vi "ATF-Pump-DI_Read.vi"(8 "error in (no error)":errorcluster, 9 "number of samples per channel":i32, 10 "DI_Task":refnum<k21>, 11 "Data FIFO Ref":T1) -> (0 "error out":errorcluster, 2 "task out":refnum<k21>)   [LabVIEW 2022 SP3]
uses:
  RT Controls/ATF-Pump-Data FIFO.ctl
  <vilib>/Platform/TimedLoop/XDataNode/timing_clust.ctl
  <vilib>/Platform/TimedLoop/XDataNode/nitl_modes.ctl
  <vilib>/Platform/TimedLoop/XDataNode/wakeup.ctl
  <vilib>/DAQmx/read.llb/DAQmx Read (Digital 1D Wfm NChan NSamp).vi
  <vilib>/DAQmx/miscellaneous.llb/DAQmx Fill In Error Info.vi
  <vilib>/Waveform/DTblOps.llb/DTbl Digital to Boolean Array.vi
  <vilib>/platform/TimedLoop/XDataNode/XDataNode.xnode
  <vilib>/Platform/TimedLoop/XDataNode/XDNodeRunTimeDep.lvlib
panel:
  out "overflow?":bool
  out "x-y":u32
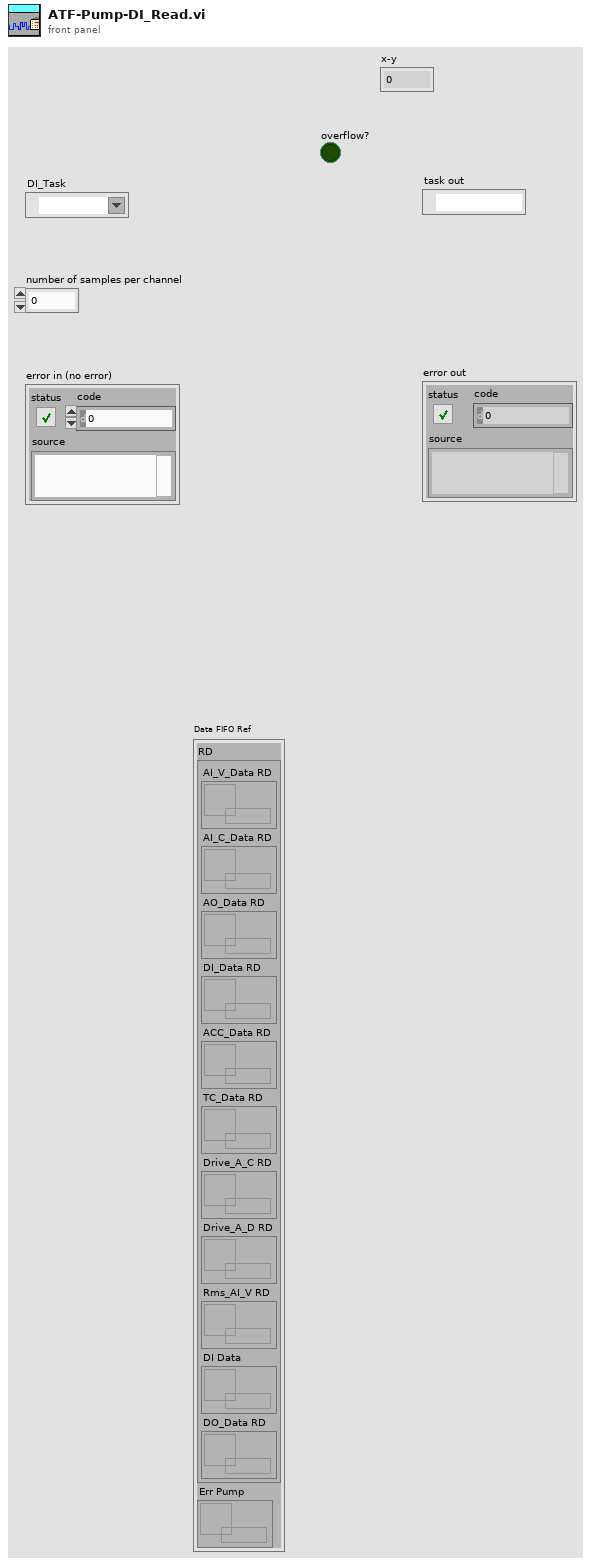
[diagram p1: front panel]
types:
  T1 = typedef "ATF-Pump-Data FIFO.ctl" = cluster{"RD":cluster{"AI_V_Data RD":refnum<queue>, "AI_C_Data RD":refnum<queue>, "AO_Data RD":refnum<queue>, "DI_Data RD":refnum<queue>, "ACC_Data RD":refnum<queue>, "TC_Data RD":refnum<queue>, "Drive_A_C RD":refnum<queue>, "Drive_A_D RD":refnum<queue>, "Rms_AI_V RD":refnum<queue>, "DI Data":refnum<queue>, "DO_Data RD":refnum<queue>}, "Err Pump":refnum<queue>}
  T2 = typedef "XDNodeRunTimeDep.lvlib/timing_clust.ctl" = cluster{"Expected End [f-1]":u64, "Actual End [f-1]":u64, "Finished Late? [f-1]":bool, "Expected End [i-1]":u64, "Actual End [i-1]":u64, "Finished Late? [i-1]":bool, "Expected Start [i]":u64, "Actual Start [i]":u64, "Expected Start [f]":u64, "Actual Start [f]":u64, "Source Name":string, "Structure Name":string, "Period":i64, "Deadline":i64, "Offset":i64, "Start":i64, "Priority":i32, "Timeout":i32, "Mode":T3, "Wakeup Reason":T4, "Error":errorcluster, "Source Type":string, "Secondary Source Type":string, "Global End Time":u64, "Global Start Time":u64, "Frame Duration":u64, "Iteration Duration":u64, "Assigned CPU":i32, "I/O Scan Engine Mode":u32}
  T3 = typedef "XDNodeRunTimeDep.lvlib/nitl_modes.ctl" = enum32{"No Change", "Process missed periods, maintain original phase", "Discard missed periods, maintain original phase", "Process missed periods, ignore original phase", "Discard missed periods, ignore original phase"}
  T4 = typedef "XDNodeRunTimeDep.lvlib/wakeup.ctl" = enum32{"Normal", "Aborted", "Asynchronous wakeup", "Timing source error", "Timed loop error", "Timeout"}
  T5 = enum16{"AI C", "AI V", "AO", "DI", "DO", "TC", "ACC", "RT PMP", "DR A"}
  T6 = enum16{"Init", "Read 'All'", "Read 'n'", "Read '1'", "Write '1'", "Write 'n'", "Write 'All'"}
  T7 = cluster{"Start DAQ":bool, "Stop DAQ":bool, "RT Stop":bool, "RT Exit":bool, "Start Seq":bool}
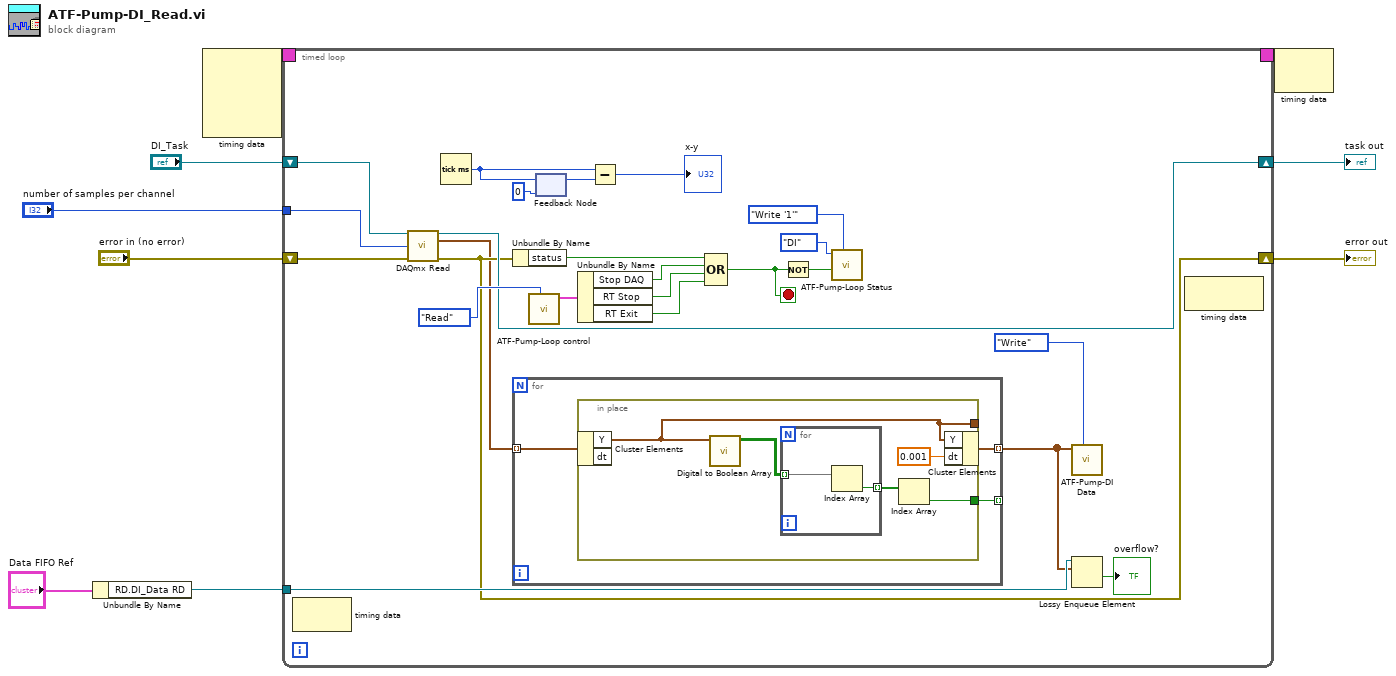
[diagram p0: block diagram]
diagram:
  n1 = Unbundle By Name("Data FIFO Ref") -> ("RD.DI_Data RD"=w3:refnum<queue>)
  n2 = node-c288() -> (w2:T2)  [unwired: 4 in]
  n3 = timed-loop {
    tunnel: "number of samples per channel" -> [w10]
    tunnel: w3 -> [w16]
    shift-right: [w18] -> w6
    shift-left: "DI_Task" -> [w32]
    shift-right: [w14] -> w5
    shift-left: "error in (no error)" -> [w31]
    timing: w2 -> [_]
    timing-out: [_] -> w1
    stop <- w33 stop-if-true
    n4 = node-c288() -> ()  [unwired: 1 in, 1 out]
    n5 = call-poly <vilib>:"DAQmx Read.vi"("task/channels in"=w32, "number of samples per channel"=w10, "error in"=w31) -> ("task out"=w18:refnum<k21>, "data"=w13:digitalwaveform[], "error out"=w14:errorcluster)  [unwired: 10 in]
    n6 = Tick Count (ms)() -> (millisecond timer value=w22:u32)
    n7 = Unbundle By Name(w14) -> ("status"=w30:bool)
    n8 = for {
      tunnel: w13 -> [w37] mode=indexing
      tunnel: [w38] -> _ mode=indexing
      tunnel: [w36] -> w12 mode=indexing
      n9 = in-place {
        in-place-border: [w39] -> w38
        in-place-border: [w40] -> _
        n10 = in-place-cluster #1(w37) -> ("Y"=w40:digitaldata)  [unwired: 1 out]
        n11 = call-poly <vilib>:"Digital to Boolean Array.vi"("digital data"=w40) -> ("boolean array"=w42:bool[][])  [unwired: 9 in, 1 out]
        n12 = for {
          tunnel: w42 -> [w45] mode=indexing
          tunnel: [w44] -> w43 mode=indexing
          n13 = Index Array(array=w45) -> (element=w44:bool)  [unwired: 1 in]
        }
        n14 = Index Array(array=w43) -> (element=w39:bool)  [unwired: 1 in]
        n15 = in-place-cluster #1("Y"=w40, "dt"=0.001) -> (w36:digitalwaveform)
      }
    }
    n16 = call "ATF-Pump-Loop control.vi"("Action"=enum16{"Init", "Write", "Read"}."Read") -> ("Loop Control out"=w25:T7)  [unwired: 9 in, 1 out]
    n17 = feedback-in #2(w22) -> ()
    n18 = feedback #2(u32 0 ("millisecond timer value")) -> (w21:u32)
    n19 = Unbundle By Name(w25) -> ("Stop DAQ"=w29:bool, "RT Stop"=w28:bool, "RT Exit"=w27:bool)
    n20 = Subtract(x=w22, y=w21) -> (x-y=→"x-y":u32)
    n21 = Compound Arithmetic op=OR(w30, w29, w28, w27) -> (w33:bool)
    n22 = Not(x=w33) -> (.not. x?=w23:bool)
    n23 = call "ATF-Pump-Loop Status.vi"("Option"=T6."Write '1'", "Status"=w23, "Loop"=T5."DI") -> ()  [unwired: 6 in, 3 out]
    n24 = call "ATF-Pump-DI Data.vi"("Enum"=enum16{"Write", "Read"}."Write", "In_DI data"=w12) -> ()  [unwired: 9 in, 1 out]
    n25 = Lossy Enqueue Element(queue=w16, element=w12) -> (overflow?=→"overflow?":bool)  [unwired: 1 in, 3 out]
    n26 = node-c288() -> ()  [unwired: 1 in, 1 out]
  }
  "task out" <- w6
  "error out" <- w5
  n27 = node-c288(w1) -> ()  [unwired: 1 out]
